vi "Write Data.vi"(8 "error in (no error)":errorcluster, 9 "Publication Time":timestamp, 10 "Value":variant, 11 "PersistToDiskTransport In":refnum<class "PersistToDiskTransport.lvclass">) -> (0 "error out":errorcluster, 3 "PersistToDiskTransport Out":refnum<class "PersistToDiskTransport.lvclass">)   [LabVIEW 2017, in "Transport.lvlib" / "PersistToDiskTransport.lvclass"]
doc: "<License>\nCopyright © 2017 Composed Systems, LLC | All rights reserved\nwww.composed.io\n\nAuthor: Ethan Stern <ethan.stern@composed.io>\n\nThis software is provided \"AS IS\" WITHOUT WARRANTIES, either express or implied, AND IS FOR EDUCATIONAL PURPOSES ONLY.\n</License>"
uses:
  PersistToDiskTransport.lvclass
  PersistToDiskTransport.lvclass/PersistToDiskTransport.ctl
  gpm_packages/@cs/variant/Source/Format Type String.vi
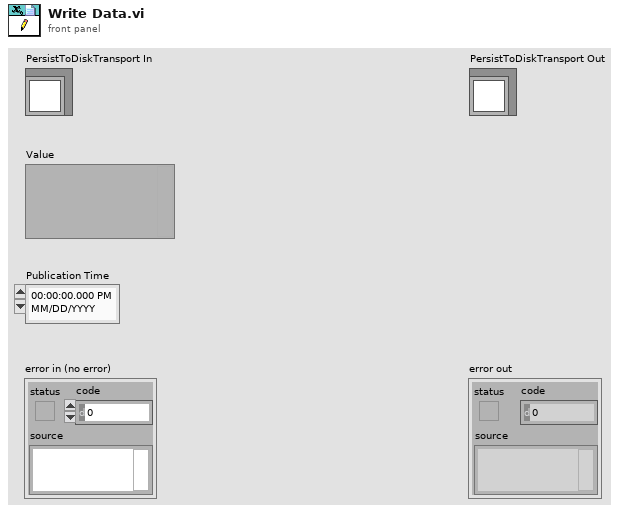
[diagram p1: front panel]
types:
  T1 = cluster{"Datum Name":string, "type string":i16[], "data string":string, "Publication Time":timestamp}
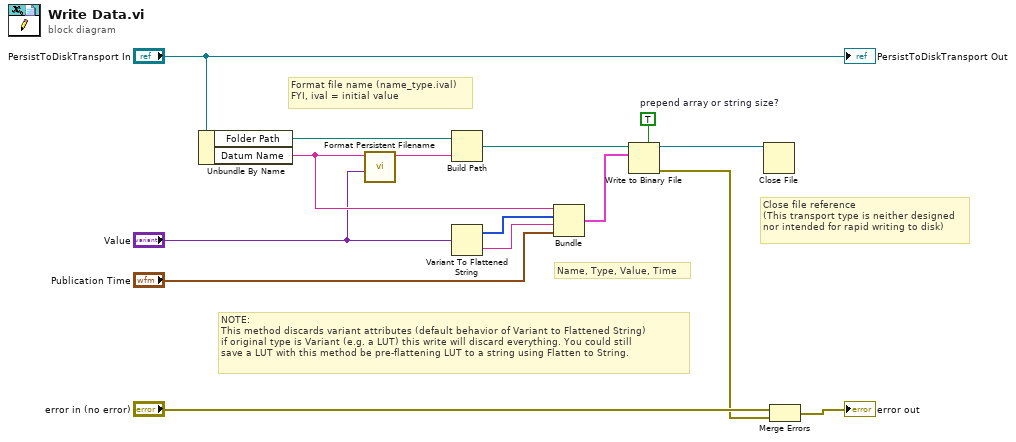
[diagram p0: block diagram]
diagram:
  w10 = TRUE  # prepend array or string size?
  # "Close file reference\n(This transport type is neither designed\nnor intended for rapid writing to disk)"
  # "Name, Type, Value, Time"
  # "NOTE:\nThis method discards variant attributes (default behavior of Variant to Flattened String)\nif original type is Variant (e.g. a LUT) this write will discard everything. You could still\nsave a LUT with this method be pre-flattening LUT to a string using Flatten to String."
  # "Format file name (name_type.ival)\nFYI, ival = initial value"
  n1 = Unbundle By Name("PersistToDiskTransport In") -> ("Folder Path"=w12:path, "Datum Name"=w7:string)
  n2 = call "Format Persistent Filename.vi"("Datum Type"="Value", "Datum Name"=w7) -> ("Filename"=w3:string)  [unwired: 9 in]
  n3 = Build Path(base path=w12, name or relative path=w3) -> (appended path=w11:path)
  n4 = Variant To Flattened String(Variant="Value") -> (data string=w8:string, 1:w9:i16[])
  n5 = Bundle("Datum Name"=w7, "type string"=w9, "data string"=w8, "Publication Time"="Publication Time") -> (w5:T1)  [unwired: 1 in]
  n6 = Write to Binary File(file (use dialog)=w11, data=w5, 5:w10) -> (refnum out=w2:refnum<file>, error out=w4:errorcluster)  [unwired: 3 in, 1 out]
  n7 = Close File(refnum=w2) -> ()  [unwired: 1 in, 2 out]
  n8 = Merge Errors("error in (no error)", w4) -> (→"error out":errorcluster)
  "PersistToDiskTransport Out" <- "PersistToDiskTransport In"
